vi "Format_Read.vi"(0 "Source Address":u32=15, 2 "Address":u32=31, 3 "Address Parity":u32=1, 5 "error in (no error)":errorcluster, 8 "CMD":u32=3) -> (15 "RFFE Read Word":u32, 19 "error out":errorcluster)   [LabVIEW 2020, in "niDigital.lvclass"]
uses:
  niDigital.lvclass
panel:
  out "x << y 1":u32
  out "x << y 6":u32
  out "x << y 9":u32
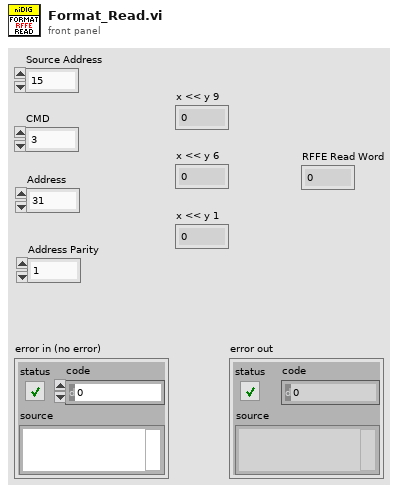
[diagram p1: front panel]
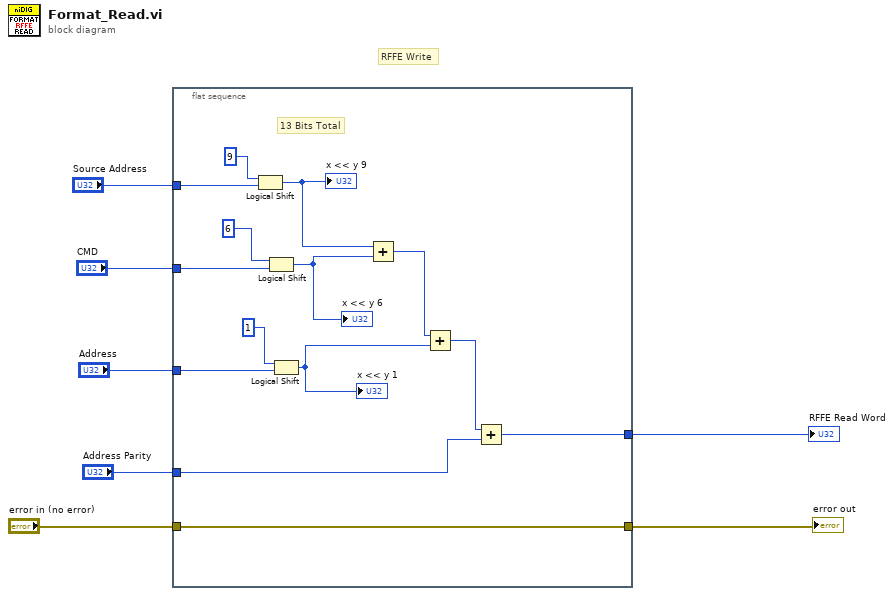
[diagram p0: block diagram]
diagram:
  # "RFFE Write"
  n1 = flat-sequence {
    tunnel: "Source Address" -> [w21]
    tunnel: "CMD" -> [w20]
    tunnel: [w19] -> w5
    tunnel: "Address" -> [w11]
    tunnel: "Address Parity" -> [w9]
    tunnel: "error in (no error)" -> [w8]
    tunnel: [w8] -> w1
    frame #0 {
      # "13 Bits Total"
      n2 = Logical Shift(y=i16 9, x=w21) -> (x << y=w17:u32)
      "x << y 9" <- w17
      n3 = Logical Shift(y=i16 6, x=w20) -> (x << y=w13:u32)
      "x << y 6" <- w13
      n4 = Logical Shift(y=i16 1, x=w11) -> (x << y=w10:u32)
      "x << y 1" <- w10
      n5 = Add(x=w17, y=w13) -> (x+y=w16:u32)
      n6 = Add(x=w16, y=w10) -> (x+y=w15:u32)
      n7 = Add(x=w15, y=w9) -> (x+y=w19:u32)
    }
  }
  "RFFE Read Word" <- w5
  "error out" <- w1
